vi "find_roi_centroid.vi"(8 "Error In":errorcluster, 10 "ROI Descriptor":T1 {"Contours"."Type" items=["No Selection", "Point", "Line", "Rectangle", "Oval", "Polygon", "Freehand Region", "Annulus", "Unused2", "Unused3", "Broken Line", "Freehand Line", "Rotated Rectangle"]}, 11 "Image Src":T2) -> (0 "error out":errorcluster, 2 "Y Centroid":sgl, 3 "X Centroid":sgl)   [LabVIEW 2019]
uses:
  <vilib>/vision/Image Controls.llb/IMAQ Image.ctl
  <vilib>/vision/NI_Vision_Development_Module.lvlib
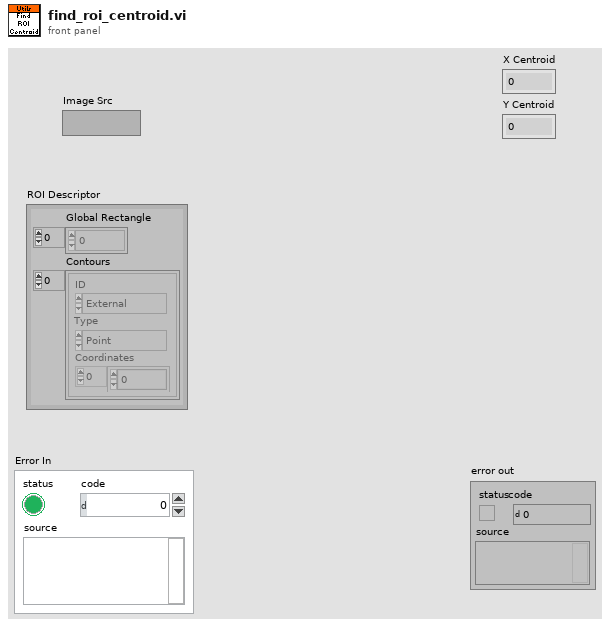
[diagram p1: front panel]
types:
  T1 = typedef "ROI Descriptor" = cluster{"Global Rectangle":i32[], "Contours":cluster{"ID":enum32{"External", "Internal"}, "Type":u32, "Coordinates":i32[]}[]}
  T2 = typedef "IMAQ Image.ctl" = refnum<image>
  T3 = typedef "Image Type" = u32
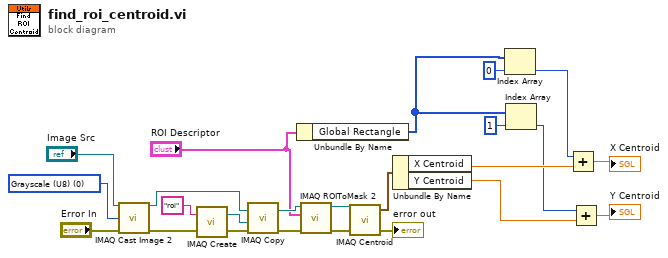
[diagram p0: block diagram]
diagram:
  w23 = T3 0 items=["Grayscale (U8)", "Grayscale (I16)", "Grayscale (SGL)", "Complex (CSG)", "RGB (U32)", "HSL (U32)", "RGB (U64)", "Grayscale (U16)"] ("Image Type")
  n1 = call "IMAQ Cast Image 2"("Image Src"="Image Src", "Image Type"=w23, "error in (no error)"="Error In") -> ("Image Dst Out"=w18:T2, "error out"=w17:errorcluster)  [unwired: 11 in]
  n2 = call "IMAQ Create"("Image Name"="roi", "error in (no error)"=w17) -> ("New Image"=w19:T2, "error out"=w20:errorcluster)  [unwired: 3 in]
  n3 = call "IMAQ Copy"("error in (no error)"=w20, "Image Dst"=w19, "Image Src"=w18) -> ("error out"=w15:errorcluster, "Image Dst Out"=w14:T2)  [unwired: 3 in]
  n4 = Unbundle By Name("ROI Descriptor") -> ("Global Rectangle"=w8:i32[])
  n5 = call "IMAQ ROIToMask 2"("error in (no error)"=w15, "ROI Descriptor"="ROI Descriptor", "Image"=w14) -> ("error out"=w16:errorcluster, "Image Out"=w11:T2)  [unwired: 6 in, 1 out]
  n6 = call "IMAQ Centroid"("error in (no error)"=w16, "Image"=w11) -> ("error out"=→"error out":errorcluster, "Centroid"=w13:cluster{"X Centroid":sgl, "Y Centroid":sgl})  [unwired: 2 in]
  n7 = Unbundle By Name(w13) -> ("X Centroid"=w3:sgl, "Y Centroid"=w1:sgl)
  n8 = Index Array(array=w8, index=0) -> (element=w4:i32)
  n9 = Index Array(array=w8, index=1) -> (element=w2:i32)
  n10 = Add(x=w4, y=w3) -> (x+y=→"X Centroid":sgl)
  n11 = Add(x=w2, y=w1) -> (x+y=→"Y Centroid":sgl)
